vi "SP Initialize Trace Orientation.vi"(8 "error in (no error)":errorcluster, 10 "CH Controls":T1[](array[typedef]) {"Traces"."Reference" format="%#.2g"; "Traces"."Display Data" items=["Data", "Memory", "Data/Memory"]; "Traces"."Format" items=["Log Mag", "Phase", "Expanded Phase", "Delay", "Smith", "Polar", "Lin Mag", "SWR", "Loss", "Real", "Imaginary"]; "Traces"."Scale" min=0.001 step=1.0 format="%#.2g"; "Traces"."Position" min=0.0 max=10.0; "Frequency"."Stop" format="%.3g"; "Frequency"."Start" format="%.3g"}, 11 "Plots Tab Control":refnum<vi>) -> (0 "error out":errorcluster)   [LabVIEW 2011]
uses:
  TypeDefs/SP Display Plot Controls Cluster.ctl
  TypeDefs/SP Frequency Units.ctl
  TypeDefs/SP Marker Cluster.ctl
  TypeDefs/SP Marker Type.ctl
  TypeDefs/SP Display Trace Controls.ctl
  TypeDefs/SP Display Format.ctl
  TypeDefs/SP Display Data.ctl
panel:
  # "Div"
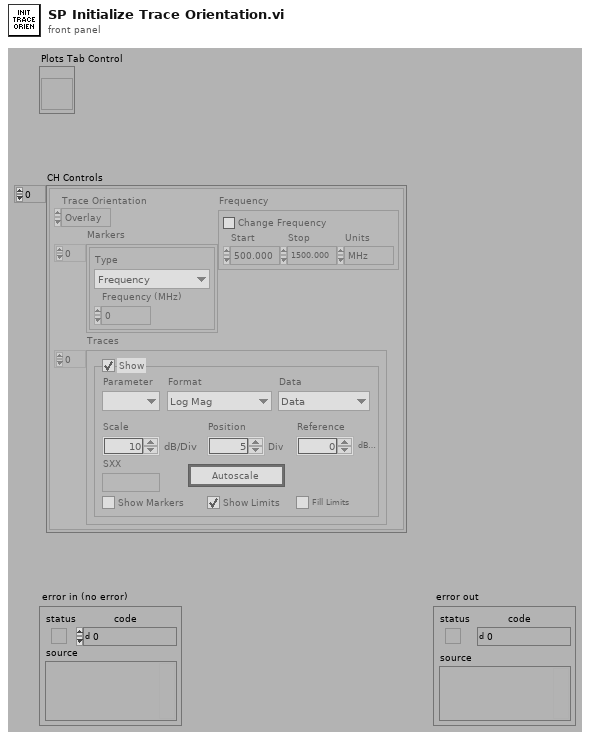
[diagram p1: front panel]
types:
  T1 = typedef "SP Display Plot Controls Cluster.ctl" = cluster{"Trace Orientation":enum32{"Overlay", "Split"}, "Frequency":cluster{"Change Frequency":bool, "Start":dbl, "Stop":dbl, "Units":T2}, "Markers":T3[], "Traces":T5[]}
  T2 = typedef "SP Frequency Units.ctl" = enum16{"Hz", "kHz", "MHz", "GHz", "Points"}
  T3 = typedef "SP Marker Cluster.ctl" = cluster{"Type":T4, "Frequency (MHz)":dbl}
  T4 = typedef "SP Marker Type.ctl" = enum16{"Frequency", "Trace Maximum", "Trace Minimum", "Limit Maximum", "Limit Minimum"}
  T5 = typedef "SP Display Trace Controls.ctl" = cluster{"Trace On":bool, "Measure":i32, "Format":T6, "Autoscale":bool, "Reference":dbl, "\nRefUnit":string, "Position":dbl, "Scale":dbl, "ScaleUnit":string, "LimitOn":bool, "LimitFill":bool, "Display Data":T7, "Show Markers":bool, "SXX":string}
  T6 = typedef "SP Display Format.ctl" = i32
  T7 = typedef "SP Display Data.ctl" = u16
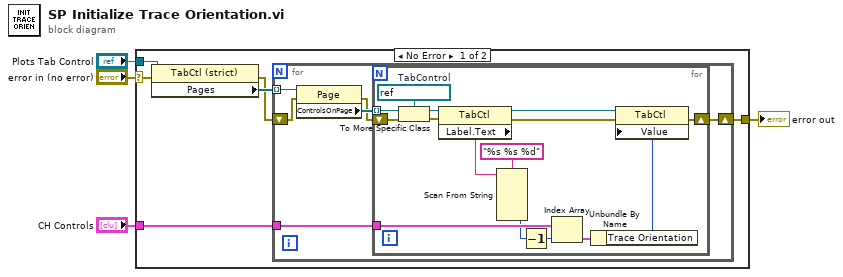
[diagram p0: block diagram]
diagram:
  n1 = case shown="No Error" "error in (no error)" {
    selector: "error in (no error)" -> [w5 w32]
    tunnel: "Plots Tab Control" -> [w10 _]
    tunnel: "CH Controls" -> [w9 _]
    tunnel: [w6 w32] -> w2
    frame No Error {
      n2 = property class="TabCtl (strict)"(reference=w10, error in=w5) -> (error out=w7:errorcluster, "Pages"=w8:refnum<vi>[])  [unwired: 1 out]
      n3 = for {
        tunnel: w9 -> [w14]
        tunnel: w8 -> [w16] mode=indexing
        shift-right: [w13] -> w6
        shift-left: w7 -> [w12]
        n4 = property class="Page"(reference=w16, error in=w12) -> (error out=w11:errorcluster, "ControlsOnPage"=w15:refnum<vi>[])  [unwired: 1 out]
        n5 = for {
          tunnel: w15 -> [w29] mode=indexing
          tunnel: w14 -> [w25]
          shift-right: [w21] -> w13
          shift-left: w11 -> [w20]
          w31 = refnum<vi> refnum  # TabControl
          n6 = To More Specific Class(target class=w31, reference=w29, error in=w20) -> (specific class reference=w30:refnum<vi>, error out=w19:errorcluster)
          n7 = property class="TabCtl"(reference=w30, error in=w19) -> (reference out=w26:refnum<vi>, error out=w18:errorcluster, "Label.Text"=w27:string)
          n8 = Scan From String(format string="%s %s %d", input string=w27) -> (output 3=w24:i32)  [unwired: 2 in, 8 out]
          n9 = Decrement(x=w24) -> (x-1=w17:i32)
          n10 = Index Array(array=w25, index=w17) -> (element=w23:T1)
          n11 = Unbundle By Name(w23) -> ("Trace Orientation"=w22:enum32{"Overlay", "Split"})
          n12 = property class="TabCtl"(reference=w26, error in=w18, "Value"=w22) -> (error out=w21:errorcluster)  [unwired: 1 out]
        }
      }
    }
    frame Error {
    }
  }
  "error out" <- w2
